vi "Open Child.vi"(8 "error in (no error)":errorcluster, 11 "TCP Server in":refnum<class "TCP Server.lvclass">) -> (0 "error out":errorcluster, 3 "TCP Server out":refnum<class "TCP Server.lvclass">)   [LabVIEW 2020, in "Stream-TCP.lvlib" / "TCP Server.lvclass"]
uses:
  TCP Server.lvclass
  <vilib>/ErrorRing/Error Ring.xnode
  <vilib>/IlluminatedG/lv-stream/Endpoint/Endpoint.lvclass
  C:/Program Files (x86)/National Instruments/LabVIEW 2020/vi.lib/IlluminatedG/lv-stream/Endpoint/Endpoint.lvclass
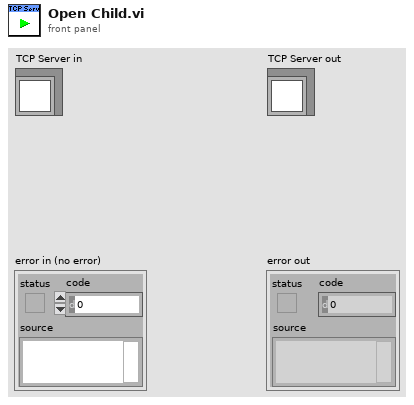
[diagram p1: front panel]
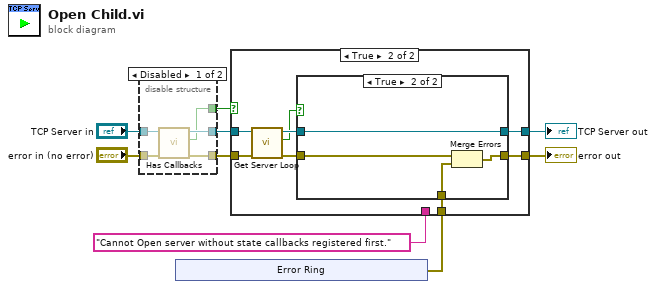
[diagram p0: block diagram]
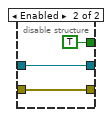
[diagram p2: hidden frame]
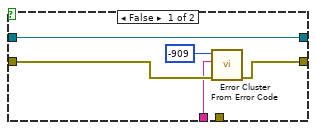
[diagram p3: hidden frame]
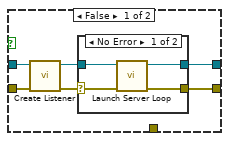
[diagram p4: hidden frame]
diagram:
  n1 = disable-structure shown="Disabled" {
    disable-tunnel: "TCP Server in" -> [w14 w16]
    disable-tunnel: [w13 w16] -> w8
    disable-tunnel: [w12 w15] -> w7
    disable-tunnel: [w11 TRUE ("Has Callbacks")] -> w6
    disable-tunnel: "error in (no error)" -> [w10 w15]
    frame Disabled {
      n2 = call <vilib>:"Has Callbacks.vi"("error in (no error)"=w10, "Endpoint in"=w14) -> ("error out"=w12:errorcluster, "Has Callbacks"=w11:bool, "Endpoint out"=w13:refnum<class "TCP Server.lvclass">)  [unwired: 7 in]
    }
    frame Enabled {
    }
  }
  n3 = xnode "Error Ring"() -> ("error out"=w4:errorcluster)
  n4 = case shown="True" w6 {
    tunnel: w8 -> [w18 w30]
    tunnel: w7 -> [w22 w29]
    tunnel: [w18 w25] -> w5
    tunnel: [w19 w24] -> w2
    tunnel: w4 -> [_ w23]
    tunnel: "Cannot Open server without state callbacks registered first." -> [w20 _]
    frame False {
      n5 = call <vilib>:"Error Cluster From Error Code.vi"("error in (no error)"=w22, "error message (\"\")"=w20, "error code (0)"=-909) -> ("error out"=w19:errorcluster)  [unwired: 6 in]
    }
    frame True {
      n6 = call "Get Server Loop.vi"("error in (no error)"=w29, "TCP Server in"=w30) -> ("error out"=w27:errorcluster, "Server Loop"=w26:bool, "TCP Server out"=w28:refnum<class "TCP Server.lvclass">)  [unwired: 7 in]
      n7 = case shown="True" w26 {
        tunnel: w28 -> [w36 w46]
        tunnel: w27 -> [w35 w45]
        tunnel: [w32 w46] -> w25
        tunnel: [w31 w44] -> w24
        tunnel: w23 -> [_ w43]
        frame False {
          n8 = call "Create Listener.vi"("error in (no error)"=w35, "TCP Server in"=w36) -> ("error out"=w34:errorcluster, "TCP Server out"=w33:refnum<class "TCP Server.lvclass">)  [unwired: 8 in]
          n9 = case shown="No Error" w34 {
            selector: w34 -> [w39 w41]
            tunnel: w33 -> [w40 w42]
            tunnel: [w38 w42] -> w32
            tunnel: [w37 w41] -> w31
            frame No Error {
              n10 = call "Launch Server Loop.vi"("error in (no error)"=w39, "TCP Server in"=w40) -> ("error out"=w37:errorcluster, "TCP Server out"=w38:refnum<class "TCP Server.lvclass">)  [unwired: 8 in]
            }
            frame Error {
            }
          }
        }
        frame True {
          n11 = Merge Errors(w45, w43) -> (w44:errorcluster)
        }
      }
    }
  }
  "error out" <- w2
  "TCP Server out" <- w5
